vi "Cálculos não uniforme.vi"(0 "Tag":string, 1 "point_data":T1, 2 "Dados in":T3, 3 "Infos para processamento in":T2={"Diâmetro do furo [mm]"=1.4, "Diâmetro da linha média [mm]"=5.0, "IncF"=0.2, "Módulo de elasticidade [GPa]"=207.0, "Módulo de Poisson"=0.3, "Tipo de roseta utilizada"=enum."Tipo A", "Método de análise"=enum."Simplificado 2008", "Pfinal"=0.3, "Parar auto."=TRUE}) -> (5 "point_data-out":T1, 6 "Resultados médios":string[][](array[string]), 7 "Resultados":dbl[][](array[numeric]))   [LabVIEW 2016]
uses:
  Controles/p,q, t, a e b.ctl
  Controles/Infos para processamento.ctl
  StressCalculations/point_data.ctl
  Report/report_mods.ctl
  <vilib>/Analysis/baseanly.llb/Mean (DBL).vi
  <vilib>/gmath/NI_Gmath.lvlib
  <vilib>/Analysis/NI_AALBase.lvlib
panel:
  out "Convergência":cluster{dbl[], dbl[]}[](graph) caption="Combinação de deformações"
  out "Stress":cluster{"z":dbl[], dbl[]}[](graph) caption="Combinação de deformações"
  out "CombDef":cluster{"z":dbl[], dbl[]}[](graph) caption="Combinação de deformações"
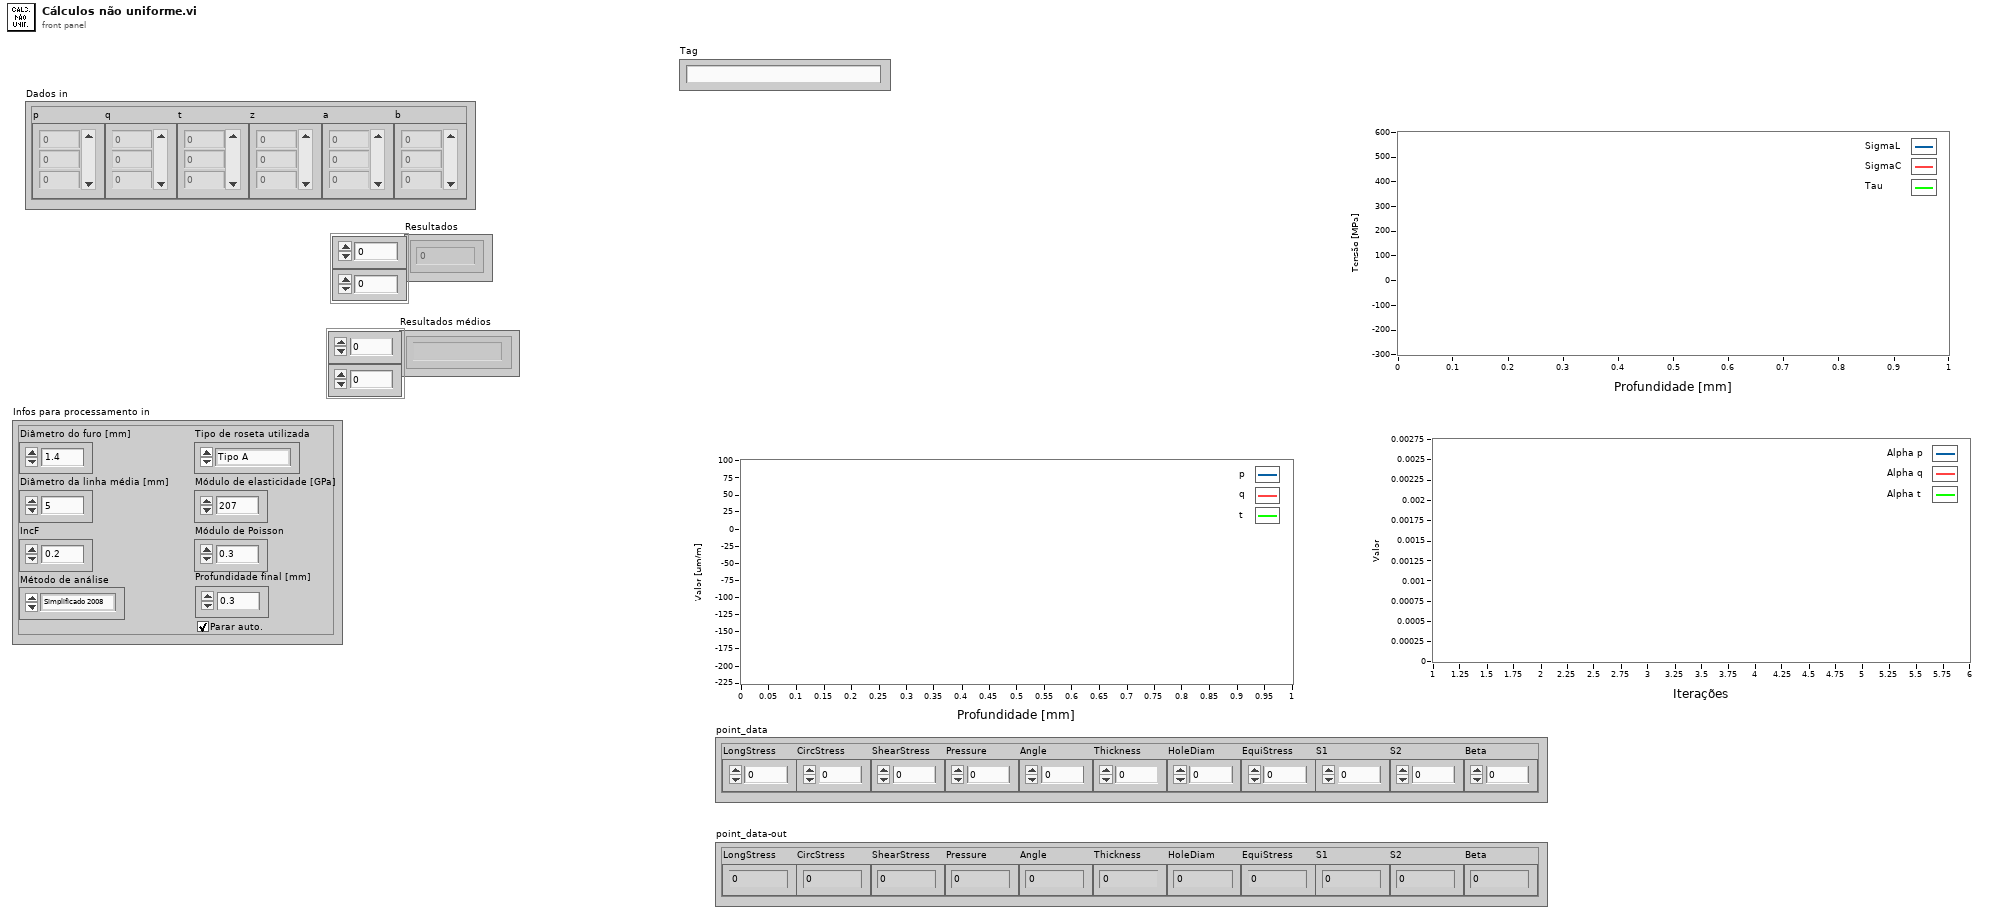
[diagram p1: front panel]
types:
  T1 = typedef "point_data.ctl" = cluster{"LongStress":dbl, "CircStress":dbl, "ShearStress":dbl, "Pressure":dbl, "Angle":dbl, "Thickness":dbl, "HoleDiam":dbl, "EquiStress":dbl, "S1":dbl, "S2":dbl, "Beta":dbl}
  T2 = typedef "Infos para processamento.ctl" = cluster{"Diâmetro do furo [mm]":dbl, "Diâmetro da linha média [mm]":dbl, "IncF":dbl, "Módulo de elasticidade [GPa]":dbl, "Módulo de Poisson":dbl, "Tipo de roseta utilizada":enum16{"Tipo A", "Tipo B", "Tipo C"}, "Método de análise":enum16{"Não uniforme 2013", "Simplificado 2013", "Simplificado 2008"}, "Pfinal":dbl, "Parar auto.":bool}
  T3 = typedef "p,q, t, a e b.ctl" = cluster{"p":dbl[], "q":dbl[], "t":dbl[], "z":dbl[], "a":dbl[], "b":dbl[]}
  T4 = typedef "report_mods.ctl" = enum16{"Init", "Table", "Graph", "TablefromGraph", "End"}
  T5 = typedef "Matrizes não uniforme.ctl" = cluster{"aT":dbl[][], "bT":dbl[][], "aTa":dbl[][], "bTb":dbl[][]}
  T6 = typedef "Resultados não uniformes.ctl" = cluster{"P":dbl[], "Q":dbl[], "T":dbl[], "P rms":dbl, "Q rms":dbl, "T rms":dbl}
  T7 = cluster{string, "Convergência":refnum<vi>, "string":string[]}
  T8 = cluster{string, "Stress":refnum<vi>, "string":string[]}
  T9 = cluster{string, "CombDef":refnum<vi>, "string":string[]}
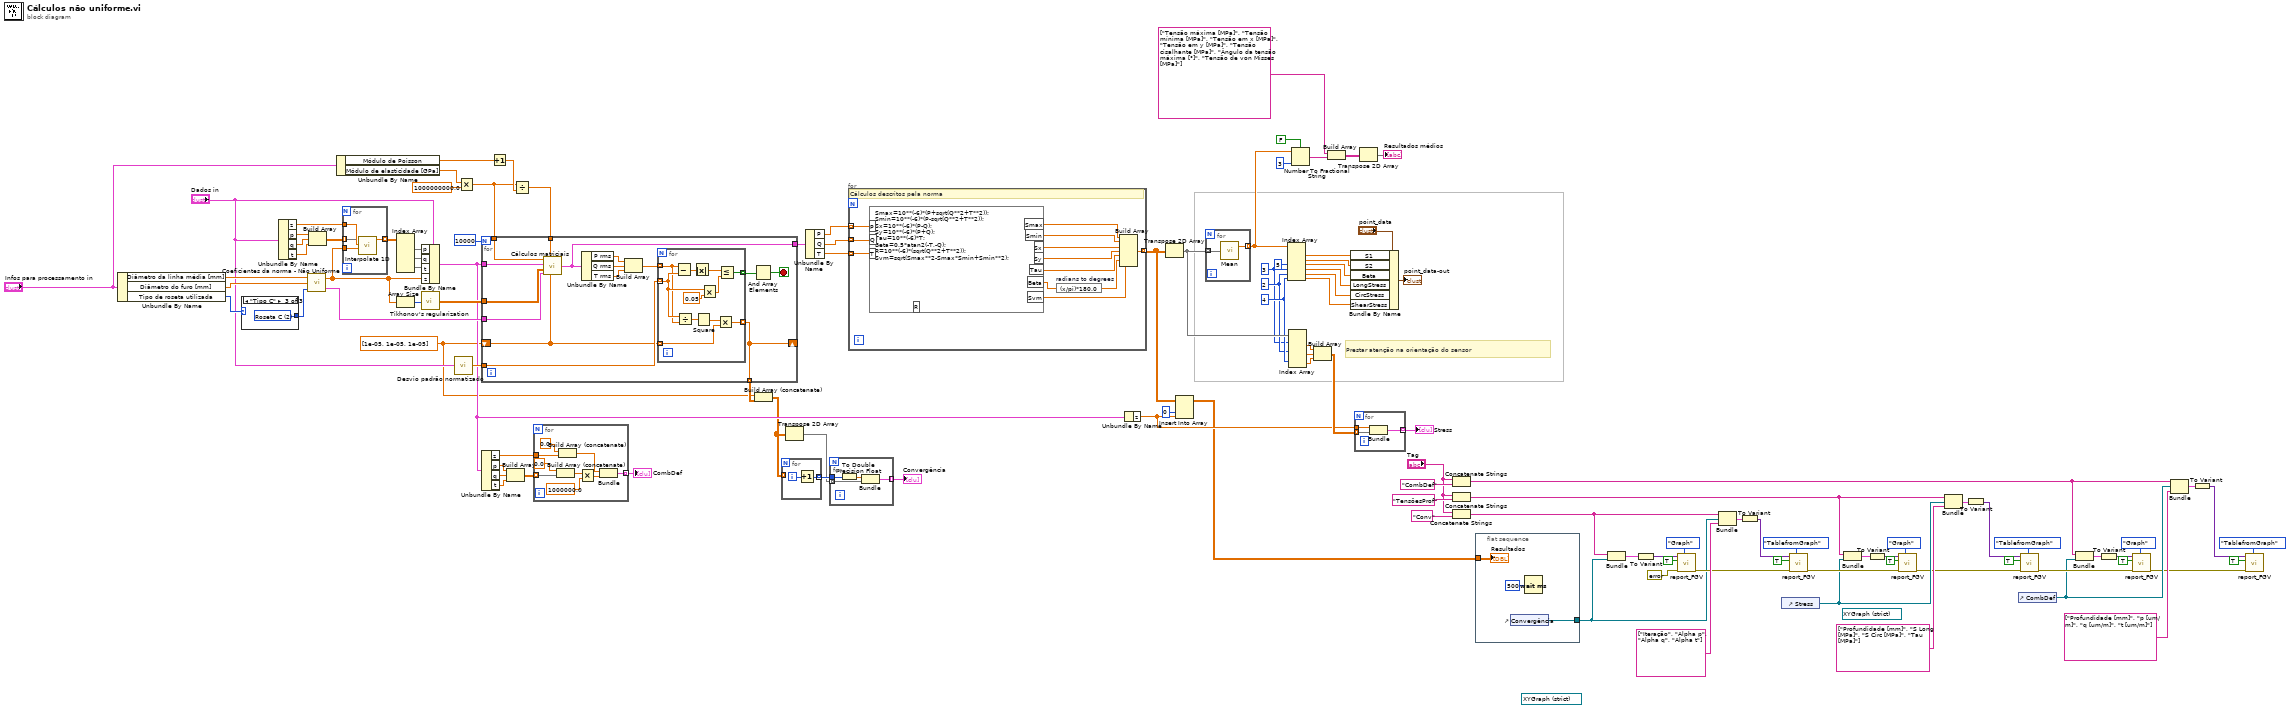
[diagram p0: block diagram]
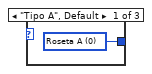
[diagram p2: hidden frame]
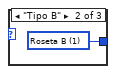
[diagram p3: hidden frame]
diagram:
  (unwired) refnum<vi> refnum ("Stress")
  (unwired) refnum<vi> refnum ("Convergência")
  w55 = 4 ("index")
  w54 = 2 ("index")
  w53 = 3 ("index")
  w70 = dbl[] [1e-05, 1e-05, 1e-05] ("Coeficientes de controle")
  # "Prestar atenção na orientação do sensor"
  n1 = Unbundle By Name("Infos para processamento in") -> ("Diâmetro da linha média [mm]"=w98:dbl, "Diâmetro do furo [mm]"=w97:dbl, "Tipo de roseta utilizada"=w96:enum16{"Tipo A", "Tipo B", "Tipo C"})
  n2 = case shown="\"Tipo C\"" w96 {
    tunnel: [w117 w118 w119] -> w95
    frame "Tipo A", Default {
      w117 = u16 0 items=["Roseta A", "Roseta B", "Roseta C"] ("Tipo de roseta")
    }
    frame "Tipo B" {
      w118 = u16 1 items=["Roseta A", "Roseta B", "Roseta C"] ("Tipo de roseta")
    }
    frame "Tipo C" {
      w119 = u16 2 items=["Roseta A", "Roseta B", "Roseta C"] ("Tipo de roseta")
    }
  }
  n3 = Unbundle By Name("Dados in") -> ("z"=w116:dbl[], "p"=w115:dbl[], "q"=w114:dbl[], "t"=w113:dbl[])
  n4 = call "Coeficientes da norma - Não Uniforme.vi"("Tipo de roseta"=w95, "Diâmetro do furo"=w97, "Diâmetro da roseta"=w98) -> ("Matrizes"=w103:T5, "Vetor das medidas"=w83:dbl[])
  n5 = Build Array(w115, w114, w113) -> (w112:dbl[][])
  n6 = Unbundle By Name("Infos para processamento in") -> ("Módulo de Poisson"=w93:dbl, "Módulo de elasticidade [GPa]"=w92:dbl)
  n7 = for {
    tunnel: w116 -> [w123]
    tunnel: w83 -> [w122]
    tunnel: w112 -> [w121] mode=indexing
    tunnel: [w120] -> w111 mode=indexing
    n8 = call <vilib>:"Interpolate 1D.vi"("xi"=w122, "X"=w123, "Y"=w121) -> ("yi"=w120:dbl[])  [unwired: 6 in, 2 out]
  }
  n9 = Index Array(array=w111) -> (element #1=w110:dbl[], element #2=w109:dbl[], element #3=w108:dbl[])  [unwired: 6 in]
  n10 = Array Size(array=w83) -> (size(s)=w107:i32)
  n11 = call "Tikhonov's regularization.vi"("Ordem"=w107) -> ("Matriz de regularização"=w104:dbl[][])
  n12 = Bundle By Name(cluster="Dados in", "p"=w110, "q"=w109, "t"=w108, "z"=w83) -> (w77:T3)
  n13 = call "Desvio padrão normatizado.vi"("Dados out"="Dados in") -> ("Desvios das deformações"=w101:dbl[])
  n14 = Multiply(x=w92, y=1000000000.0) -> (x*y=w91:dbl)
  n15 = Unbundle By Name(w77) -> ("z"=w73:dbl[], "p"=w76:dbl[], "q"=w75:dbl[], "t"=w74:dbl[])
  n16 = Increment(x=w93) -> (x+1=w105:dbl)
  n17 = Build Array(w76, w75, w74) -> (w72:dbl[][])
  n18 = Divide(x=w91, y=w105) -> (x/y=w102:dbl)
  n19 = for {
    N: 10000 -> [_]
    tunnel: w104 -> [w134]
    tunnel: w77 -> [w138]
    tunnel: w103 -> [w137]
    tunnel: w102 -> [w136]
    tunnel: w91 -> [w135]
    shift-right: [w124] -> _
    shift-left: w70 -> [w126]
    tunnel: w101 -> [w129]
    tunnel: [w125] -> w99
    tunnel: [w124] -> w71 mode=indexing
    stop <- w127 stop-if-true
    n20 = call "Cálculos matriciais.vi"("Coeficientes de controle"=w126, "G"=w136, "Matrizes"=w137, "Matriz de regularização"=w134, "Dados in"=w138, "E"=w135) -> ("Resultados"=w125:T6)
    n21 = Unbundle By Name(w125) -> ("P rms"=w133:dbl, "Q rms"=w132:dbl, "T rms"=w131:dbl)
    n22 = Build Array(w133, w132, w131) -> (w130:dbl[])
    n23 = for {
      tunnel: w130 -> [w145] mode=indexing
      tunnel: w129 -> [w146] mode=indexing
      tunnel: [w147] -> w128 mode=indexing
      tunnel: w126 -> [w142] mode=indexing
      tunnel: [w141] -> w124 mode=indexing
      n24 = Subtract(x=w145, y=w146) -> (x-y=w149:dbl)
      n25 = Divide(x=w146, y=w145) -> (x/y=w144:dbl)
      n26 = Absolute Value(x=w149) -> (abs(x)=w139:dbl)
      n27 = Square(x=w144) -> (x^2=w143:dbl)
      n28 = Multiply(x=w146, y=0.05) -> (x*y=w140:dbl)
      n29 = Multiply(x=w143, y=w142) -> (x*y=w141:dbl)
      n30 = Less Or Equal?(x=w139, y=w140) -> (x <= y?=w147:bool)
    }
    n31 = And Array Elements(Boolean array=w128) -> (logical AND=w127:bool)
  }
  n32 = for {
    tunnel: w73 -> [w154]
    tunnel: w72 -> [w157] mode=indexing
    tunnel: [w158] -> w43 mode=indexing
    n33 = Build Array (concatenate)(0.0, w157) -> (w153:dbl[])
    n34 = Build Array (concatenate)(0.0, w154) -> (w150:dbl[])
    n35 = Multiply(x=w153, y=1000000.0) -> (x*y=w151:dbl[])
    n36 = Bundle(w150, w151) -> (w158:cluster{dbl[], dbl[]})  [unwired: 1 in]
  }
  "CombDef" <- w43
  n37 = Build Array (concatenate)(w70, w71) -> (w32:dbl[][])
  n38 = for {
    tunnel: w32 -> [_] mode=indexing
    tunnel: [w159] -> w31 mode=indexing
    i -> [w160]
    n39 = Increment(x=w160) -> (x+1=w159:i32)
  }
  n40 = Transpose 2D Array(2D array=w32) -> (transposed array=w30:dbl[][])
  n41 = Unbundle By Name(w99) -> ("P"=w80:dbl[], "Q"=w79:dbl[], "T"=w78:dbl[])
  n42 = for {
    tunnel: w31 -> [w164]
    tunnel: w30 -> [w163] mode=indexing
    tunnel: [w162] -> w29 mode=indexing
    n43 = To Double Precision Float(number=w164) -> (double precision float=w161:dbl[])
    n44 = Bundle(w161, w163) -> (w162:cluster{dbl[], dbl[]})  [unwired: 1 in]
  }
  "Convergência" <- w29
  n45 = for {
    tunnel: w80 -> [w167] mode=indexing
    tunnel: w79 -> [w166] mode=indexing
    tunnel: w78 -> [w165] mode=indexing
    tunnel: [w174] -> w81 mode=indexing
    # "Cálculos descritos pela norma"
    n46 = formula code="Smax=10**(-6)*(P+sqrt(Q**2+T**2));\nSmin=10**(-6)*(P-sqrt(Q**2+T**2));\nSx=10**(-6)*(P-Q);\nSy=10**(-6)*(P+Q);\nTau=10**(-6)*T;\nBeta=0.5*atan2(-T,-Q);\nR=10**(-6)*(sqrt(Q**2+T**2));\nSvm=sqrt(Smax**2-Smax*Smin+Smin**2);"("P"=w167, "Q"=w166, "T"=w165) -> ("Smax"=w173:dbl, "Smin"=w172:dbl, "Sx"=w169:dbl, "Sy"=w176:dbl, "Tau"=w175:dbl, "Beta"=w171:dbl, "Svm"=w168:dbl)  [unwired: 1 out]
    n47 = expression code="(x/pi)*180.0" "radians to degrees"(w171) -> (w170:dbl)
    n48 = Build Array(w173, w172, w169, w176, w175, w170, w168) -> (w174:dbl[])
  }
  n49 = Unbundle By Name(w77) -> ("z"=w64:dbl[])
  n50 = Transpose 2D Array(2D array=w81) -> (transposed array=w69:dbl[][])
  n51 = Insert Into Array(array=w81, index (col)=0 ("disabled index (col)"), new element=w64) -> (w2:dbl[][])  [unwired: 1 in]
  n52 = for {
    tunnel: w69 -> [w178] mode=indexing
    tunnel: [w177] -> w33 mode=indexing
    n53 = call-poly <vilib>:"Mean.vi"("X"=w178) -> ("mean"=w177:dbl)  [unwired: 1 out]
  }
  n54 = Index Array(array=w33, index #3=5 ("index"), index #4=w53, index #5=w54, index #6=w55) -> (element #1=w41:dbl, element #2=w40:dbl, element #3=w38:dbl, element #4=w37:dbl, element #5=w36:dbl, element #6=w35:dbl)  [unwired: 2 in]
  n55 = Index Array(array=w69, index (row) #1=w53, index (row) #2=w54, index (row) #3=w55) -> (element #1=w68:dbl[], element #2=w67:dbl[], element #3=w66:dbl[])  [unwired: 3 in]
  n56 = Number To Fractional String(use system decimal point (T)=FALSE, number=w33, precision (6)=i16 3) -> (F-format string=w87:string[])  [unwired: 1 in]
  n57 = Build Array(w68, w67, w66) -> (w65:dbl[][])
  n58 = Build Array(string[] ["Tensão máxima [MPa]", "Tensão mínima [MPa]", "Tensão em x [MPa]", "Tensão em y [MPa]", "Tensão cisalhante [MPa]", "Ângulo da tensão máxima [°]", "Tensão de von Misses [MPa]"] ("element"), w87) -> (w85:string[][])
  n59 = Bundle By Name(cluster="point_data", "S1"=w41, "S2"=w40, "Beta"=w38, "LongStress"=w37, "CircStress"=w36, "ShearStress"=w35) -> (→"point_data-out":T1)
  n60 = for {
    tunnel: w65 -> [w180] mode=indexing
    tunnel: w64 -> [w181]
    tunnel: [w179] -> w1 mode=indexing
    n61 = Bundle("z"=w181, w180) -> (w179:cluster{"z":dbl[], dbl[]})  [unwired: 1 in]
  }
  "Stress" <- w1
  n62 = Transpose 2D Array(2D array=w85) -> (transposed array=→"Resultados médios":string[][])
  n63 = Concatenate Strings("Tag", "CombDef" ("string")) -> (w10:string)
  n64 = Concatenate Strings("Tag", "Conv" ("string")) -> (w28:string)
  n65 = Concatenate Strings("Tag", "TensõesProf" ("string")) -> (w19:string)
  n66 = flat-sequence {
    tunnel: [w184] -> w3
    tunnel: w2 -> [w183]
    frame #0 {
      n67 = control-ref of="Convergência"() -> (w184:refnum<vi>)
      n68 = Wait (ms)(milliseconds to wait=u32 500) -> ()  [unwired: 1 out]
      "Resultados" <- w183
    }
  }
  n69 = Bundle(w28, "Convergência"=w3) -> (w59:cluster{string, "Convergência":refnum<vi>})  [unwired: 1 in]
  n70 = To Variant(anything=w59) -> (Variant=w58:variant)
  n71 = call "report_FGV.vi"("report_mods"=report_mods."Graph", "Error In"=errorcluster {"status"=FALSE, "code"=0, "source"=""}, "Append?"=TRUE, "Data in"=w58) -> ("Error Out"=w24:errorcluster)  [unwired: 7 in]
  n72 = Bundle(w28, "Convergência"=w3, "string"=string[] ["Iteração", "Alpha p", "Alpha q", "Alpha t"]) -> (w23:T7)  [unwired: 1 in]
  n73 = To Variant(anything=w23) -> (Variant=w22:variant)
  n74 = control-ref of="Stress"() -> (w18:refnum<vi>)
  n75 = call "report_FGV.vi"("report_mods"=report_mods."TablefromGraph", "Error In"=w24, "Append?"=TRUE, "Data in"=w22) -> ("Error Out"=w21:errorcluster)  [unwired: 7 in]
  n76 = Bundle(w19, "Stress"=w18) -> (w51:cluster{string, "Stress":refnum<vi>})  [unwired: 1 in]
  n77 = To Variant(anything=w51) -> (Variant=w50:variant)
  n78 = call "report_FGV.vi"("report_mods"=report_mods."Graph", "Error In"=w21, "Append?"=TRUE, "Data in"=w50) -> ("Error Out"=w14:errorcluster)  [unwired: 7 in]
  n79 = Bundle(w19, "Stress"=w18, "string"=string[] ["Profundidade [mm]", "S Long [MPa]", "S Circ [MPa]", "Tau [MPa]"]) -> (w20:T8)  [unwired: 1 in]
  n80 = To Variant(anything=w20) -> (Variant=w13:variant)
  n81 = control-ref of="CombDef"() -> (w9:refnum<vi>)
  n82 = call "report_FGV.vi"("report_mods"=report_mods."TablefromGraph", "Error In"=w14, "Append?"=TRUE, "Data in"=w13) -> ("Error Out"=w12:errorcluster)  [unwired: 7 in]
  n83 = Bundle(w10, "CombDef"=w9) -> (w48:cluster{string, "CombDef":refnum<vi>})  [unwired: 1 in]
  n84 = To Variant(anything=w48) -> (Variant=w49:variant)
  n85 = call "report_FGV.vi"("report_mods"=report_mods."Graph", "Error In"=w12, "Append?"=TRUE, "Data in"=w49) -> ("Error Out"=w5:errorcluster)  [unwired: 7 in]
  n86 = Bundle(w10, "CombDef"=w9, "string"=string[] ["Profundidade [mm]", "p [um/m]", "q [um/m]", "t [um/m]"]) -> (w11:T9)  [unwired: 1 in]
  n87 = To Variant(anything=w11) -> (Variant=w4:variant)
  n88 = call "report_FGV.vi"("report_mods"=report_mods."TablefromGraph", "Error In"=w5, "Append?"=TRUE, "Data in"=w4) -> ()  [unwired: 7 in, 1 out]
